vi "Strip_VI_and_Exe_from_Path.vi"(1 "App Path":path) -> (0 "App Path out":path)   [LabVIEW 2011]
doc: "This VI will allow you to find the folder where the project is currently running from. This will work for executables and for un-compiled LabView projects. This capability allows you to locate default files and folders inside of your LabView project. This is very useful for saving and loading data and configuration files in your project."
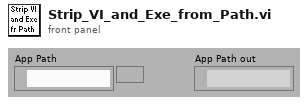
[diagram p1: front panel]
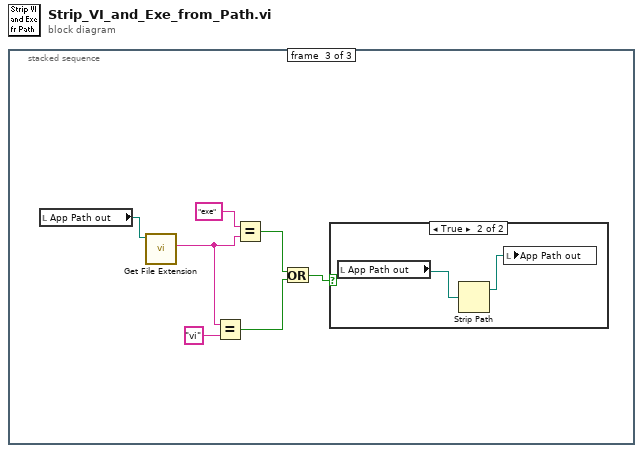
[diagram p0: block diagram]
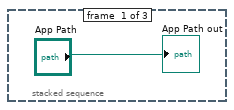
[diagram p2: hidden frame]
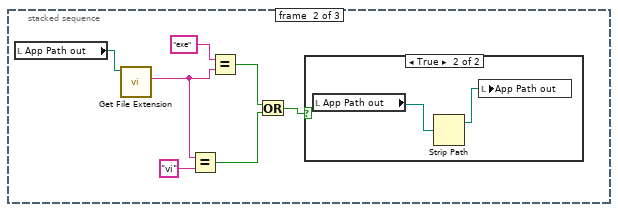
[diagram p3: hidden frame]
diagram:
  n1 = stacked-sequence {
    frame #0 {
      "App Path out" <- "App Path"
    }
    frame #1 {
      n2 = local read "App Path out"() -> (w8:path)
      n3 = call <vilib>:"Get File Extension.vi"("file"=w8) -> ("lowercase file extension"=w5:string)  [unwired: 7 in, 3 out]
      n4 = Equal?(x=w5, y="vi") -> (x = y?=w3:bool)
      n5 = Equal?(x="exe" ("y"), y=w5) -> (x = y?=w4:bool)
      n6 = Or(x=w4, y=w3) -> (x .or. y?=w2:bool)
      n7 = case shown="True" w2 {
        frame False {
        }
        frame True {
          n8 = local read "App Path out"() -> (w10:path)
          n9 = Strip Path(path=w10) -> (stripped path=w9:path)  [unwired: 1 out]
          n10 = local write "App Path out"(w9) -> ()
        }
      }
    }
    frame #2 {
      n11 = local read "App Path out"() -> (w17:path)
      n12 = call <vilib>:"Get File Extension.vi"("file"=w17) -> ("lowercase file extension"=w14:string)  [unwired: 7 in, 3 out]
      n13 = Equal?(x=w14, y="vi") -> (x = y?=w12:bool)
      n14 = Equal?(x="exe" ("y"), y=w14) -> (x = y?=w13:bool)
      n15 = Or(x=w13, y=w12) -> (x .or. y?=w11:bool)
      n16 = case shown="True" w11 {
        frame False {
        }
        frame True {
          n17 = local read "App Path out"() -> (w19:path)
          n18 = Strip Path(path=w19) -> (stripped path=w18:path)  [unwired: 1 out]
          n19 = local write "App Path out"(w18) -> ()
        }
      }
    }
  }
